vi "LINX - Digital Read N Channels.vi"() -> ()   [LabVIEW 2011, in "LMH-LINX.lvlib"]
doc: "This example demonstrates how to read N channels of digital input from a LINX device."
uses:
  vi.lib/MakerHub/LINX/LMH-LINX.lvlib
  vi.lib/MakerHub/LINX/Public/Peripherals/Digital/Digital Read N Chans.vi
panel:
  out "Values":bool[](array[boolean])
  in  "DI Channels":u8[](array[numeric])=[2, 3, 4]
  in  "Stop Button":bool
  in  "Serial Port":refnum<visa-resource-name>
  # "LINX Device Settings"
  # "Digital Read N Channel Example\n\nThis example demonstrates how to read multiple digital input channels.\n\nInstructions\n1. Select the COM Port associated with the LINX Device.\n2. Select the DI Channels to read.\n3. Click the Run Arrow."
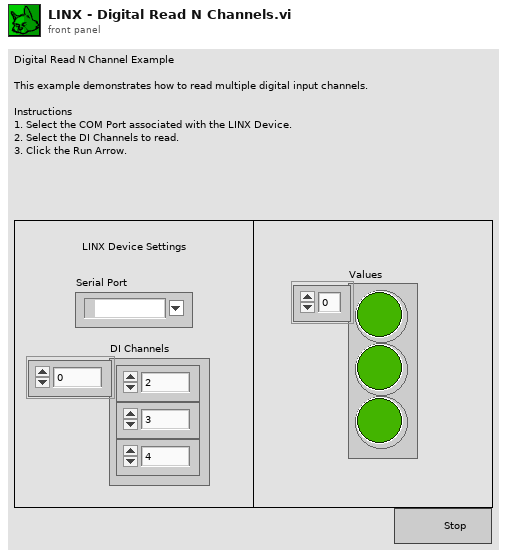
[diagram p1: front panel]
types:
  T1 = typedef "LMH-LINX.lvlib/LINX Ref.ctl" = cluster{"Platform":T2, "Interface":T3, "LINX Device Config":T4}
  T2 = typedef "LMH-LINX.lvlib/Platform.ctl" = enum16{"LINX", "myRIO"}
  T3 = typedef "LMH-LINX.lvlib/Interface.ctl" = enum16{"Serial", "TCP"}
  T4 = typedef "LMH-LINX.lvlib/Device.lvlib/LINX Device Config.ctl" = cluster{"Interface":T3, "COM Port":refnum<visa-resource-name>, "TCP Configuration":T5, "Device Family":u8, "Device ID":u8, "Device Name":string, "TCP Ref":refnum<k5>, "Channels":T6}
  T5 = typedef "LMH-LINX.lvlib/Device.lvlib/TCP Config.ctl" = cluster{"IP Address":string, "Port":u16}
  T6 = typedef "LMH-LINX.lvlib/Channels.ctl" = cluster{"DI":u8[], "DO":u8[], "AI":u8[], "AO":u8[], "PWM":u8[], "QE":u8[], "UART":u8[], "I2C 2":u8[], "SPI":u8[], "CAN":u8[], "Servo":u8[], "AI Ref (V)":dbl, "AO Ref (V)":dbl, "AO Resolution (Bits)":u8}
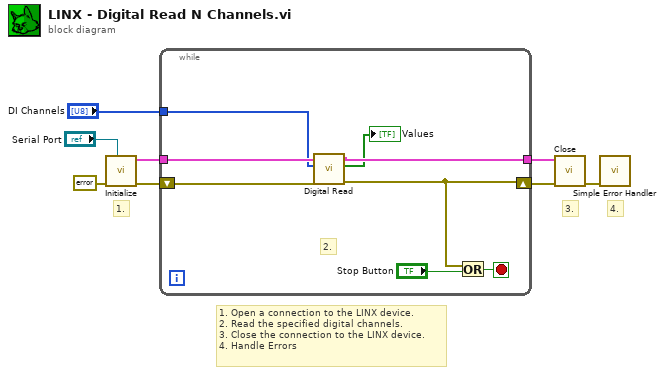
[diagram p0: block diagram]
diagram:
  # "1. Open a connection to the LINX device.\n2. Read the specified digital channels.\n3. Close the connection to the LINX device.\n4. Handle Errors"
  # "4."
  # "3."
  # "1."
  n1 = call "Initialize.vi"("Serial Port"="Serial Port", "Error In"=errorcluster {"status"=FALSE, "code"=0, "source"=""}) -> ("Error Out"=w7:errorcluster, "LINX Ref"=w8:T1)  [unwired: 7 in, 1 out]
  n2 = while {
    tunnel: w8 -> [w12]
    tunnel: [w13] -> w6
    shift-right: [w14] -> w5
    shift-left: w7 -> [w11]
    tunnel: "DI Channels" -> [w10]
    stop <- w16 stop-if-true
    # "2."
    n3 = call-poly "Digital Read.vi"("Error In"=w11, "DI Channels"=w10, "LINX Resource"=w12) -> ("Error Out"=w14:errorcluster, "Values"=→"Values":bool[], "LINX Resource"=w13:T1)  [unwired: 6 in]
    n4 = Or(x=w14, y="Stop Button") -> (x .or. y?=w16:bool)
  }
  n5 = call "Close.vi"("Error In"=w5, "LINX Resource"=w6) -> ("Error Out"=w3:errorcluster)  [unwired: 8 in, 1 out]
  n6 = call <vilib>:"Simple Error Handler.vi"("error in (no error)"=w3) -> ()  [unwired: 4 in, 5 out]
